vi "acel result.vi"(8 "Pattern amplitude":dbl, 9 "Pattern frequency (Hz)":dbl, 10 "Frecuencia de muestreo (Hz)":dbl, 11 "medidas":sgl[][](array[numeric])) -> (2 "Report":string, 3 "Calibration parameter":dbl)   [LabVIEW 2015]
uses:
  <vilib>/Analysis/5stat.llb/RMS (DBL).vi
  <vilib>/measure/madcrms.llb/Basic Averaged DC-RMS for 1 Chan.vi
  <vilib>/measure/NI_MAPro.lvlib
  <vilib>/Analysis/NI_AALPro.lvlib
  <vilib>/Analysis/NI_AALBase.lvlib
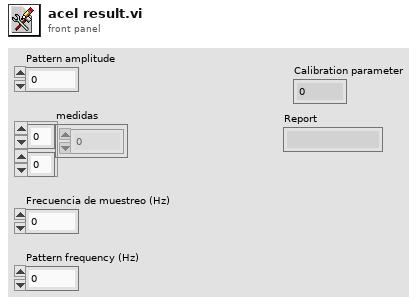
[diagram p1: front panel]
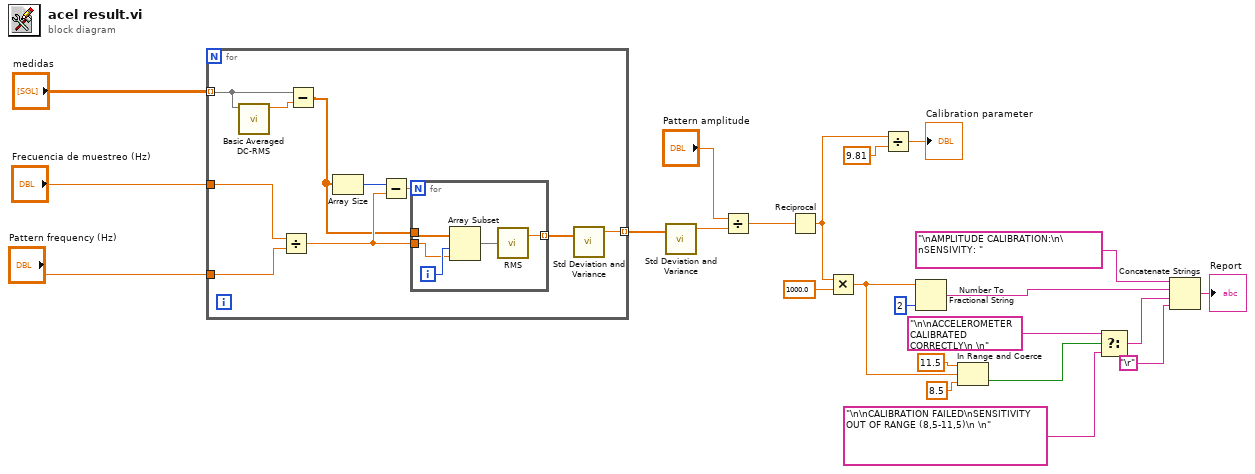
[diagram p0: block diagram]
diagram:
  n1 = for {
    tunnel: "medidas" -> [w32] mode=indexing
    tunnel: "Frecuencia de muestreo (Hz)" -> [w28]
    tunnel: "Pattern frequency (Hz)" -> [w25]
    tunnel: [w26] -> w18 mode=indexing
    n2 = call-poly <vilib>:"Basic Averaged DC-RMS.vi"("signal in"=w32) -> ("DC value"=w33:dbl)  [unwired: 7 in, 3 out]
    n3 = Divide(x=w28, y=w25) -> (x/y=w29:dbl)
    n4 = Subtract(x=w32, y=w33) -> (x-y=w24:dbl[])
    n5 = Array Size(array=w24) -> (size(s)=w30:i32)
    n6 = Subtract(x=w30, y=w29) -> (x-y=w31:dbl)
    n7 = for {
      N: w31 -> [_]
      tunnel: w29 -> [w35]
      tunnel: [w38] -> w27 mode=indexing
      tunnel: w24 -> [w37]
      i -> [w36]
      n8 = Array Subset(array=w37, index=w36, length=w35) -> (w34:dbl[])
      n9 = call-poly <vilib>:"RMS.vi"("X"=w34) -> ("rms value"=w38:dbl)  [unwired: 1 out]
    }
    n10 = call <vilib>:"Std Deviation and Variance.vi"("X"=w27) -> ("mean"=w26:dbl)  [unwired: 1 in, 2 out]
  }
  n11 = call <vilib>:"Std Deviation and Variance.vi"("X"=w18) -> ("mean"=w2:dbl)  [unwired: 1 in, 2 out]
  n12 = Divide(x="Pattern amplitude", y=w2) -> (x/y=w4:dbl)
  n13 = Reciprocal(x=w4) -> (1/x=w6:dbl)
  n14 = Multiply(x=w6, y=1000.0) -> (x*y=w9:dbl)
  n15 = Divide(x=w6, y=9.81) -> (x/y=→"Calibration parameter":dbl)
  n16 = Number To Fractional String(number=w9, precision (6)=i16 2) -> (F-format string=w13:string)  [unwired: 2 in]
  n17 = In Range and Coerce(upper limit=11.5, x=w9, lower limit=8.5) -> (In Range?=w15:bool)  [unwired: 1 out]
  n18 = Select(t="\n\nACCELEROMETER CALIBRATED CORRECTLY\n \n", s=w15, f="\n\nCALIBRATION FAILED\nSENSITIVITY OUT OF RANGE (8,5-11,5)\n \n") -> (s? t:f=w14:string)
  n19 = Concatenate Strings("\nAMPLITUDE CALIBRATION:\n\nSENSIVITY: ", w13, w14, "\r") -> (→"Report":string)
